vi "Senal_viva.vi"() -> ()   [LabVIEW 2016]
panel:
  in  "Stop Button":bool
  out "Waveform Chart":cluster{dbl, dbl, dbl, dbl}(graph)
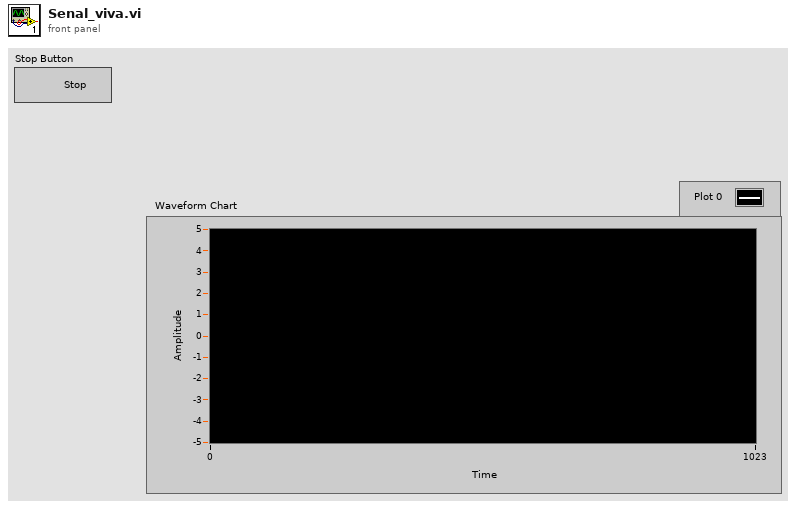
[diagram p1: front panel]
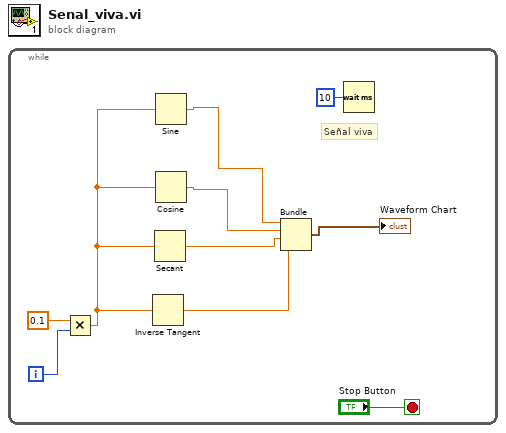
[diagram p0: block diagram]
diagram:
  n1 = while {
    i -> [w9]
    stop <- "Stop Button" stop-if-true
    # "Señal viva"
    n2 = Multiply(x=0.1, y=w9) -> (x*y=w6:dbl)
    n3 = Inverse Tangent(1:w6) -> (0:w1:dbl)
    n4 = Secant(1:w6) -> (0:w2:dbl)
    n5 = Sine(x=w6) -> (sin(x)=w3:dbl)
    n6 = Cosine(x=w6) -> (cos(x)=w4:dbl)
    n7 = Bundle(w3, w4, w2, w1) -> (→"Waveform Chart":cluster{dbl, dbl, dbl, dbl})  [unwired: 1 in]
    n8 = Wait (ms)(milliseconds to wait=u32 10) -> ()  [unwired: 1 out]
  }
